vi "validate configuration.vi"(8 "error in":errorcluster, 11 "EthernetIP configuration in":refnum<class "EIP Tags Configuration.lvclass">) -> (0 "error out":errorcluster, 3 "EthernetIP configuration out":refnum<class "EIP Tags Configuration.lvclass">)   [LabVIEW 2013, in "EIP Tags Configuration.lvclass"]
doc: "This function performs validation of the configuration. This function should be safe to call at any point and should not rely on anything in the runtime environment."
uses:
  EIP Tags Configuration.lvclass
  <vilib>/NI/Tag Bus Module Framework/module configuration/TBM module configuration.lvclass
  EIP Tags Configuration.lvclass/EIP Tags Configuration.ctl
  channel/EIP Tags Channel.lvclass/EIP Tags Channel.ctl
  channel/Read Instance ID.vi
  channel/EIP Tags Channel.lvclass
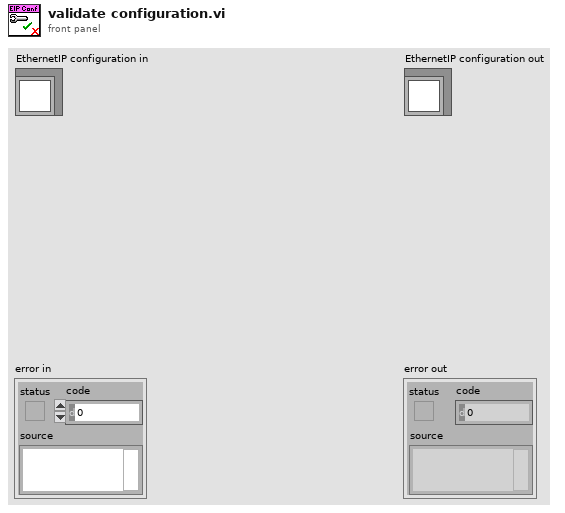
[diagram p1: front panel]
types:
  T1 = typedef "EIP Tags Configuration.lvclass/assembly definition.ctl" = cluster{"name":string, "Instance ID":u32, "Type":T2, "Size (bytes)":u32, "big endian?":bool}
  T2 = typedef "EIP Tags Configuration.lvclass/assembly type.ctl" = enum32{"Producing", "Consuming"}
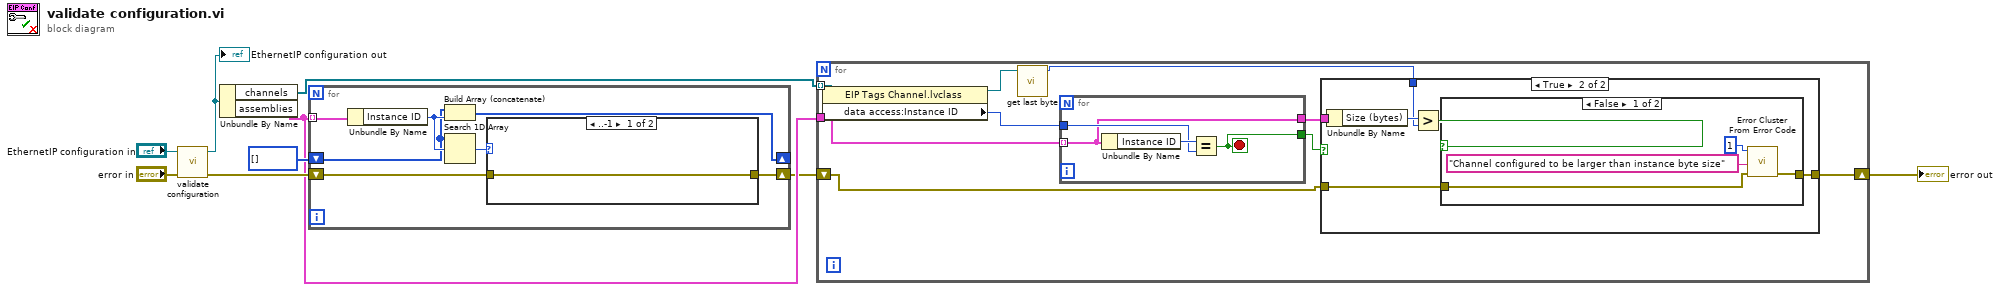
[diagram p0: block diagram]
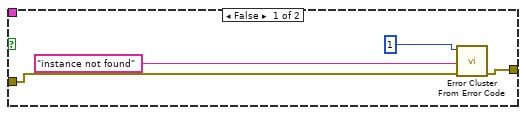
[diagram p2: hidden frame]
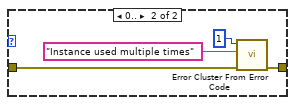
[diagram p4: hidden frame]
diagram:
  n1 = call-parent "validate configuration.vi"("error in"="error in", "configuration in"="EthernetIP configuration in") -> ("error out"=w5:errorcluster, "configuration out"=w7:refnum<class "EIP Tags Configuration.lvclass">)  [unwired: 8 in]
  "EthernetIP configuration out" <- w7
  n2 = Unbundle By Name(w7) -> ("channels"=w4:refnum<class "EIP Tags Channel.lvclass">[], "assemblies"=w3:T1[])
  n3 = for {
    tunnel: w3 -> [w16] mode=indexing
    shift-right: [w15] -> _
    shift-left: u32[] [] -> [w13]
    shift-right: [w11] -> w2
    shift-left: w5 -> [w12]
    n4 = Unbundle By Name(w16) -> ("Instance ID"=w14:u32)
    n5 = Build Array (concatenate)(w13, w14) -> (w15:u32[])
    n6 = Search 1D Array(1D array=w13, element=w14) -> (index of element=w10:i32)  [unwired: 1 in]
    n7 = case shown="..-1" w10 {
      tunnel: w12 -> [w17 w20]
      tunnel: [w17 w21] -> w11
      frame ..-1 {
      }
      frame 0.. {
        n8 = call <vilib>:"Error Cluster From Error Code.vi"("error in (no error)"=w20, "error message (\"\")"="Instance used multiple times" ("error message (\"\")"), "error code (0)"=1) -> ("error out"=w21:errorcluster)  [unwired: 6 in]
      }
    }
  }
  n9 = for {
    tunnel: w4 -> [w29] mode=indexing
    tunnel: w3 -> [w30]
    shift-right: [w23] -> w1
    shift-left: w2 -> [w24]
    n10 = property class="EIP Tags Channel.lvclass"(reference=w29) -> (reference out=w27:refnum<class "EIP Tags Channel.lvclass">, "data access:Instance ID"=w28:u32)  [unwired: 1 in, 1 out]
    n11 = call "get last byte.vi"("EthernetIP Channel in"=w27) -> ("last byte"=w22:i32)  [unwired: 10 in]
    n12 = for {
      tunnel: w30 -> [w47] mode=indexing
      tunnel: w28 -> [w48]
      tunnel: [w47] -> w25
      tunnel: [w46] -> w26
      stop <- w46 stop-if-true
      n13 = Unbundle By Name(w47) -> ("Instance ID"=w49:u32)
      n14 = Equal?(x=w49, y=w48) -> (x = y?=w46:bool)
    }
    n15 = case shown="True" w26 {
      tunnel: w25 -> [_ w40]
      tunnel: w24 -> [w33 w35]
      tunnel: [w32 w36] -> w23
      tunnel: w22 -> [_ w38]
      frame False {
        n16 = call <vilib>:"Error Cluster From Error Code.vi"("error in (no error)"=w33, "error message (\"\")"="instance not found" ("error message (\"\")"), "error code (0)"=1) -> ("error out"=w32:errorcluster)  [unwired: 6 in]
      }
      frame True {
        n17 = Unbundle By Name(w40) -> ("Size (bytes)"=w39:u32)
        n18 = Greater?(x=w39, y=w38) -> (0:w37:bool)
        n19 = case shown="False" w37 {
          tunnel: [w41 w45] -> w36
          tunnel: w35 -> [w42 w45]
          frame False {
            n20 = call <vilib>:"Error Cluster From Error Code.vi"("error in (no error)"=w42, "error message (\"\")"="Channel configured to be larger than instance byte size" ("error message (\"\")"), "error code (0)"=1) -> ("error out"=w41:errorcluster)  [unwired: 6 in]
          }
          frame True {
          }
        }
      }
    }
  }
  "error out" <- w1
